vi "Field to Current Converter.vi"(1 "Field[T]":dbl, 2 "Field constant[T/A]":dbl) -> (0 "Current[A]":dbl)   [LabVIEW 2022 SP3, in "Magnet module.lvlib"]
uses:
  Magnet module.lvlib
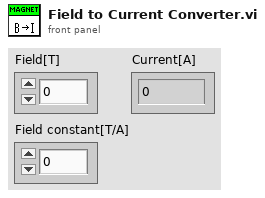
[diagram p1: front panel]
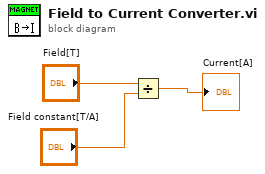
[diagram p0: block diagram]
diagram:
  n1 = Divide(x="Field[T]", y="Field constant[T/A]") -> (x/y=→"Current[A]":dbl)
